vi "纳清_第二点原始光强值写入.vi"(7 "探头":T1(ring), 8 "error in (no error)":errorcluster caption="错误输入（无错误）", 10 "数值":sgl, 11 "MB session in":refnum<class "MB_Master.lvclass">) -> (0 "error out":errorcluster caption="错误输出", 3 "MB session out":refnum<class "MB_Master.lvclass">)   [LabVIEW 2016, in "斯坦道多参数.lvlib"]
uses:
  <vilib>/Plasmionique/MB Master/MB_Master/MB_Master.lvclass
  <vilib>/Plasmionique/MB Master/MB Master.lvlib
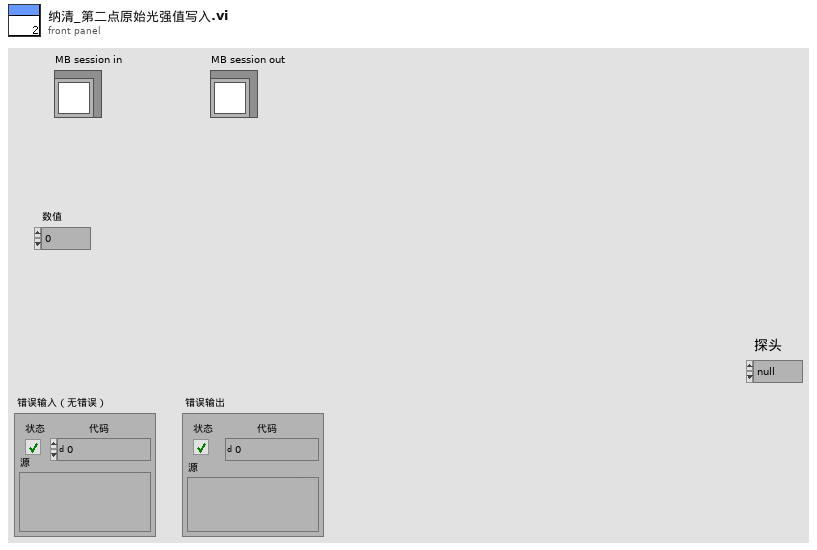
[diagram p1: front panel]
types:
  T1 = enum16{"null", "pH", "DO", "浊度", "电导率", "叶绿素a", "藻密度"}
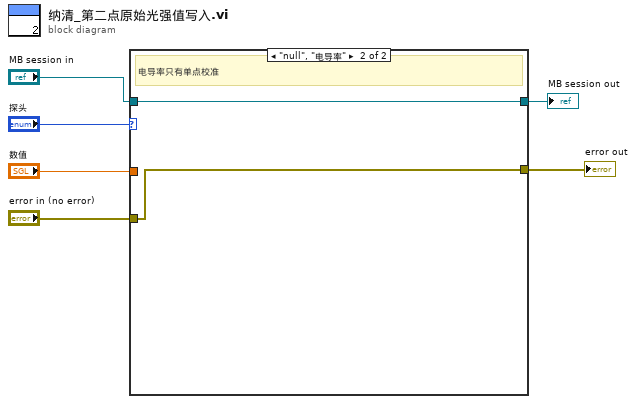
[diagram p0: block diagram]
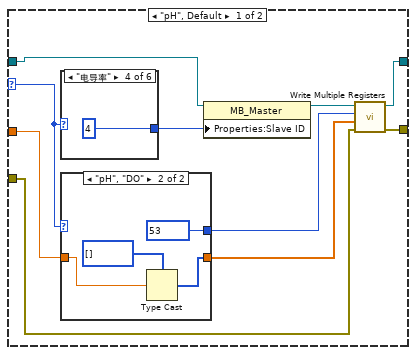
[diagram p2: hidden frame]
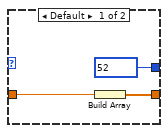
[diagram p3: hidden frame]
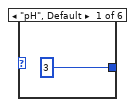
[diagram p4: hidden frame]
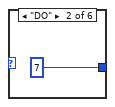
[diagram p5: hidden frame]
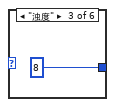
[diagram p6: hidden frame]
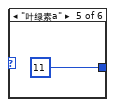
[diagram p7: hidden frame]
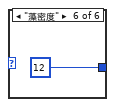
[diagram p8: hidden frame]
diagram:
  n1 = case shown="\"null\", \"电导率\"" "探头" {
    selector: "探头" -> [w7 _]
    tunnel: "error in (no error)" -> [w16 w30]
    tunnel: [w15 w30] -> w5
    tunnel: "MB session in" -> [w13 w31]
    tunnel: [w12 w31] -> w3
    tunnel: "数值" -> [w10 _]
    frame "pH", Default {
      n2 = case shown="\"电导率\"" w7 {
        tunnel: [3 7 8 4 11 12] -> w11
        frame "pH", Default {
        }
        frame "DO" {
        }
        frame "浊度" {
        }
        frame "电导率" {
        }
        frame "叶绿素a" {
        }
        frame "藻密度" {
        }
      }
      n3 = case shown="\"pH\", \"DO\"" w7 {
        tunnel: w10 -> [w19 w22]
        tunnel: [w18 w21] -> w9
        tunnel: [u16 52 ("starting address") u16 53 ("starting address")] -> w8
        frame Default {
          n4 = Build Array(w19) -> (w18:sgl[])
        }
        frame "pH", "DO" {
          n5 = Type Cast(type=u16[] [], x=w22) -> (*(type *) &x=w21:u16[])
        }
      }
      n6 = property class="MB_Master"(reference=w13, "Properties:Slave ID"=w11) -> (reference out=w14:refnum<class "MB_Master.lvclass">)  [unwired: 1 in, 1 out]
      n7 = call <vilib>:"Write Multiple Registers.vi"("error in (no error)"=w16, "values"=w9, "starting address"=w8, "MB session in"=w14) -> ("error out"=w15:errorcluster, "MB session out"=w12:refnum<class "MB_Master.lvclass">)  [unwired: 6 in]
    }
    frame "null", "电导率" {
      # "电导率只有单点校准"
    }
  }
  "error out" <- w5
  "MB session out" <- w3
